vi "Initialize.vi"(8 "error in (no error)":errorcluster, 9 "Requestor":string, 10 "Requestee":string, 11 "Mag Lab Hardware in":refnum<class "Software Lock-in.lvclass">) -> (0 "error out":errorcluster, 3 "Mag Lab Hardware out":refnum<class "Software Lock-in.lvclass">)   [LabVIEW 2015, in "Software Lock-in.lvclass"]
uses:
  Software Lock-in.lvclass
  Software Lock-in.lvclass/Software Lock-in.ctl
  Mag Lab Hardware.lvclass
  <vilib>/Analysis/NI_AALBase.lvlib
  Mag Lab Error Handler/Mag Lab Error Handler.lvclass
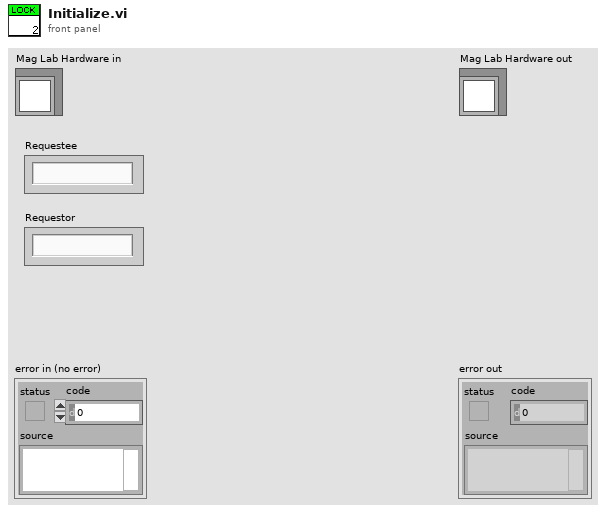
[diagram p1: front panel]
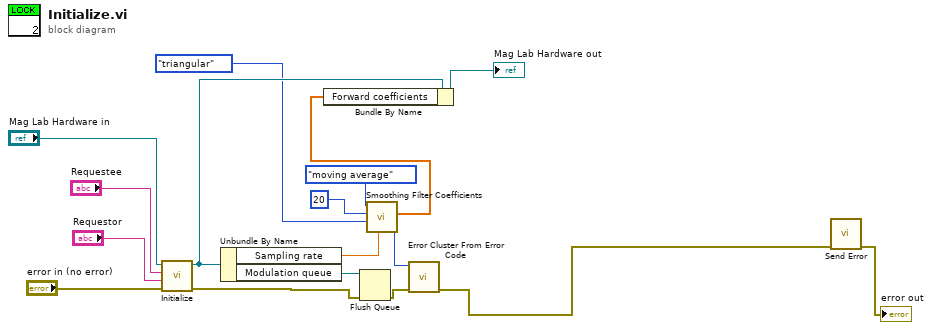
[diagram p0: block diagram]
diagram:
  n1 = call-parent "Initialize.vi"("error in (no error)"="error in (no error)", "Requestor"="Requestor", "Requestee"="Requestee", "Mag Lab Hardware in"="Mag Lab Hardware in") -> ("error out"=w6:errorcluster, "Mag Lab Hardware out"=w13:refnum<class "Software Lock-in.lvclass">)  [unwired: 6 in]
  n2 = Unbundle By Name(w13) -> ("Sampling rate"=w7:dbl, "Modulation queue"=w4:refnum<queue>)
  n3 = Flush Queue(queue=w4, error in (no error)=w6) -> (error out=w5:errorcluster)  [unwired: 2 out]
  n4 = call <vilib>:"Smoothing Filter Coefficients.vi"("fs"=w7, "shape"=enum16{"rectangular", "triangular"}."triangular", "half-width"=20, "type"=enum16{"moving average", "exponential"}."moving average") -> ("error"=w3:i32, "forward coefficients"=w8:dbl[])  [unwired: 5 in, 1 out]
  n5 = Bundle By Name(cluster=w13, "Forward coefficients"=w8) -> (→"Mag Lab Hardware out":refnum<class "Software Lock-in.lvclass">)
  n6 = call <vilib>:"Error Cluster From Error Code.vi"("error in (no error)"=w5, "error code (0)"=w3) -> ("error out"=w2:errorcluster)  [unwired: 7 in]
  n7 = call "Send Error.vi"("error in (no error)"=w2) -> ("error out"=→"error out":errorcluster)  [unwired: 9 in, 1 out]
